vi "Check Load Editor.vi"(8 "error in (no error)":errorcluster, 11 "Engine in":refnum<class "Engine.lvclass">) -> (0 "error out":errorcluster, 3 "Engine out":refnum<class "Engine.lvclass">)   [LabVIEW 2020, in "TSnax.lvlib" / "Engine.lvclass"]
uses:
  Engine.lvclass
  Engine.lvclass/Engine.ctl
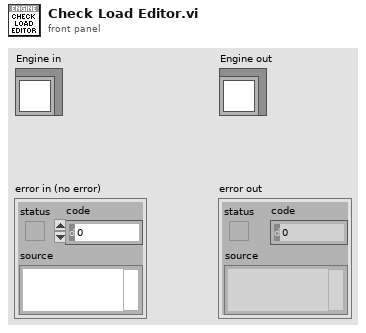
[diagram p1: front panel]
types:
  T1 = typedef "TSnax.lvlib/Engine.lvclass/TS License Type.ctl" = enum16{"Operator", "CustomEditor", "SequenceEditor"}
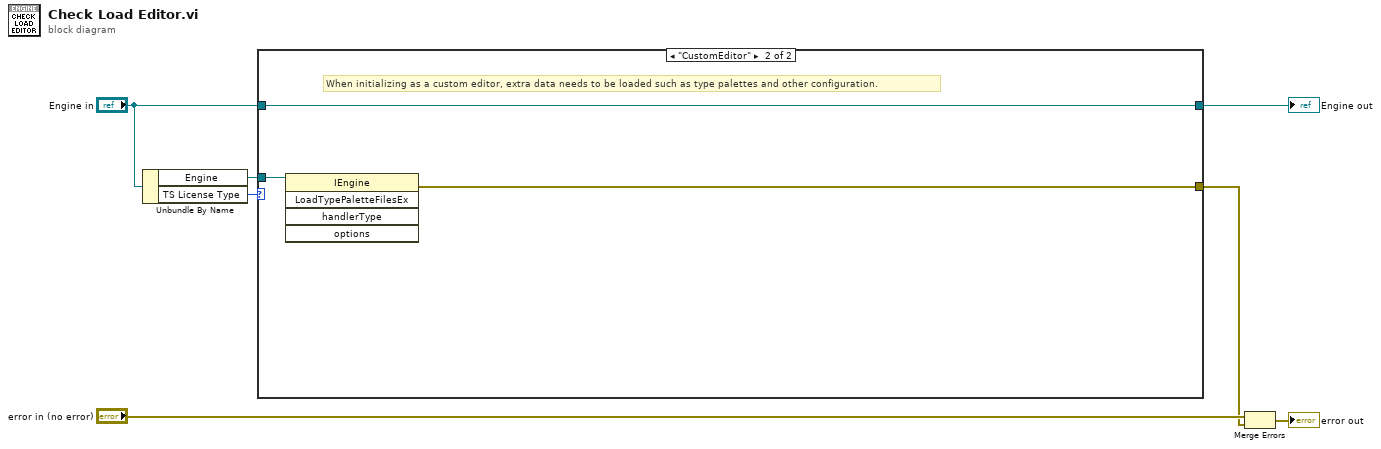
[diagram p0: block diagram]
diagram:
  n1 = Unbundle By Name("Engine in") -> ("Engine"=w4:refnum<k7>, "TS License Type"=w7:T1)
  n2 = case shown="\"CustomEditor\"" w7 {
    tunnel: "Engine in" -> [w8 w10]
    tunnel: [w8 w10] -> w5
    tunnel: w4 -> [_ w11]
    tunnel: [_ w9] -> w1
    frame Default {
    }
    frame "CustomEditor" {
      # "When initializing as a custom editor, extra data needs to be loaded such as type palettes and other configuration."
      n3 = invoke class="IEngine" method="LoadTypePaletteFilesEx"(reference=w11) -> (error out=w9:errorcluster)  [unwired: 4 in, 4 out]
    }
  }
  "Engine out" <- w5
  n4 = Merge Errors("error in (no error)", w1) -> (→"error out":errorcluster)
